vi "Robot_Disabled.vi"() -> (3 "Robot Disabled":bool)   [LabVIEW 2023]
doc: "Return TRUE if robot is disabled."
uses:
  <vilib>/Rock Robotics/WPI/DriverStation/WPI_DriverStationRobotMode2.ctl
  Robot Global Data.vi
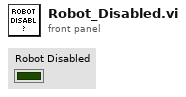
[diagram p1: front panel]
types:
  T1 = typedef "WPI_DriverStationRobotMode2.ctl" = enum16{"Autonomous Disabled", "Autonomous Enabled", "Teleop Disabled", "Teleop Enabled", "Disconnected", "Finish", "Test Disabled", "Test Enabled", "Emergency Stopped"}
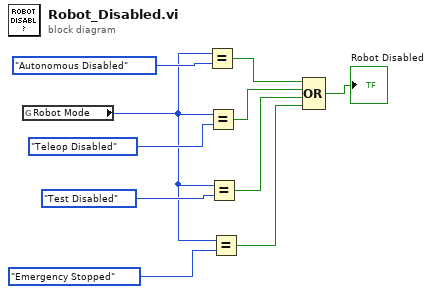
[diagram p0: block diagram]
diagram:
  n1 = global read "Robot Global Data.vi" "Robot Mode"() -> (w2:T1)
  n2 = Equal?(x=w2, y=WPI_DriverStationRobotMode2."Autonomous Disabled") -> (x = y?=w9:bool)
  n3 = Equal?(x=w2, y=WPI_DriverStationRobotMode2."Teleop Disabled") -> (x = y?=w10:bool)
  n4 = Equal?(x=w2, y=WPI_DriverStationRobotMode2."Test Disabled") -> (x = y?=w4:bool)
  n5 = Equal?(x=w2, y=WPI_DriverStationRobotMode2."Emergency Stopped") -> (x = y?=w1:bool)
  n6 = Compound Arithmetic op=OR(w9, w10, w4, w1) -> (→"Robot Disabled":bool)
